vi "DKGSM_old.vi"(9 "input":T1, 10 "State":string) -> (2 "DKGSMOutput":T2)   [LabVIEW 2015]
uses:
  Typedefs/DKGSMOut.ctl
  Typedefs/DKGSMin.ctl
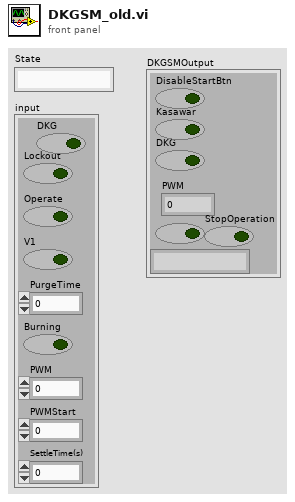
[diagram p1: front panel]
types:
  T1 = typedef "DKGSMin.ctl" = cluster{"Lockout":bool, "Operate":bool, "V1":bool, "PurgeTime":dbl, "Burning":bool, "PWM":i32, "PWMStart":i32, "SettleTime(s)":dbl, "DKG":bool}
  T2 = typedef "DKGSMOut.ctl" = cluster{"DisableStartBtn":bool, "Kasawar":bool, "DKG":bool, "PWM":i32, "Purge":bool, "Opis":string, "StopOperation":bool}
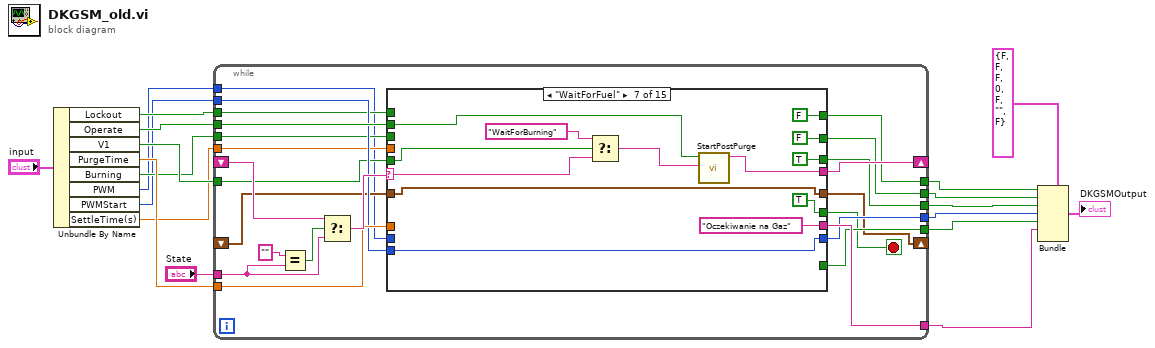
[diagram p0: block diagram]
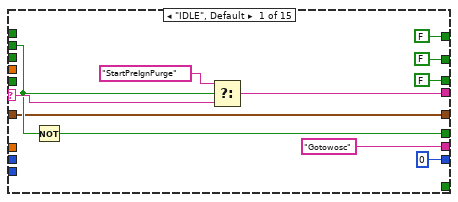
[diagram p2: hidden frame]
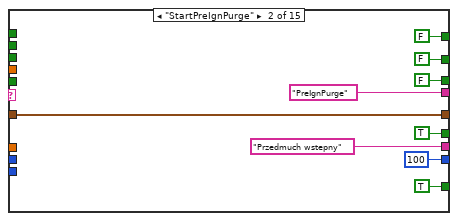
[diagram p3: hidden frame]
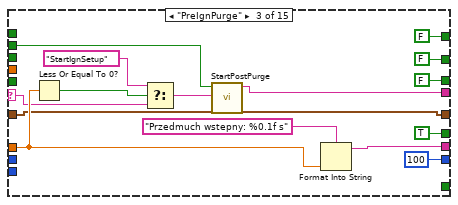
[diagram p4: hidden frame]
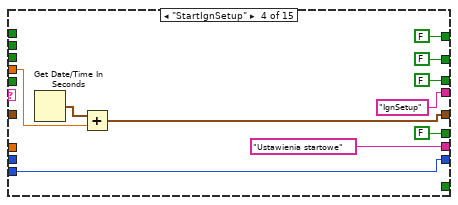
[diagram p5: hidden frame]
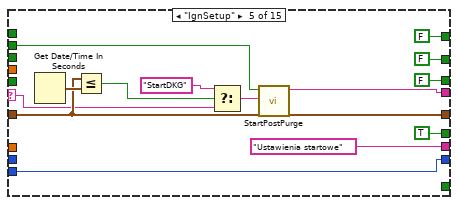
[diagram p6: hidden frame]
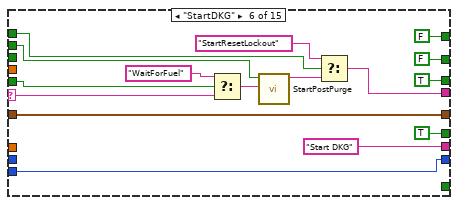
[diagram p7: hidden frame]
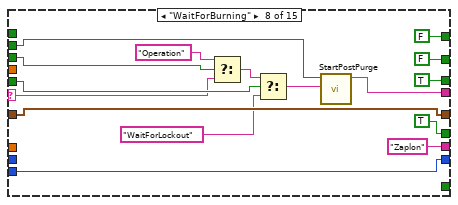
[diagram p8: hidden frame]
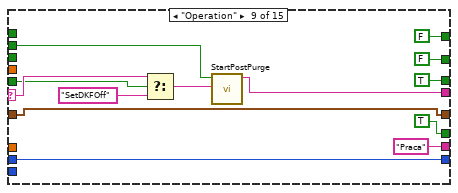
[diagram p9: hidden frame]
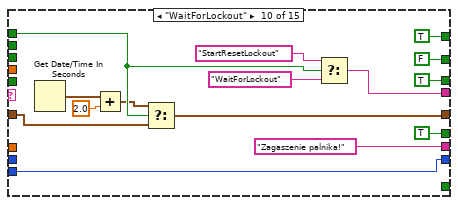
[diagram p10: hidden frame]
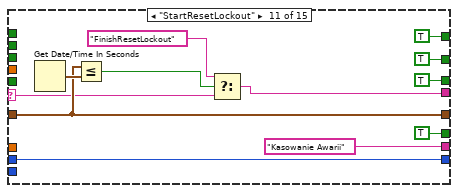
[diagram p11: hidden frame]
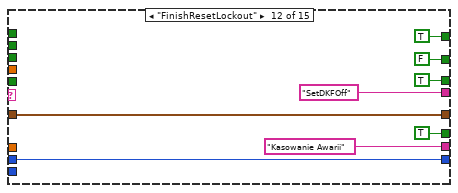
[diagram p12: hidden frame]
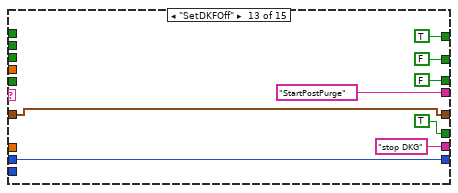
[diagram p13: hidden frame]
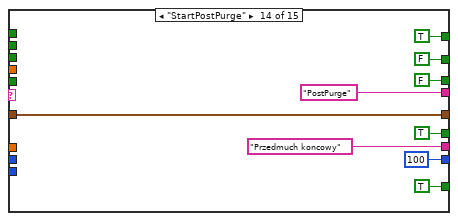
[diagram p14: hidden frame]
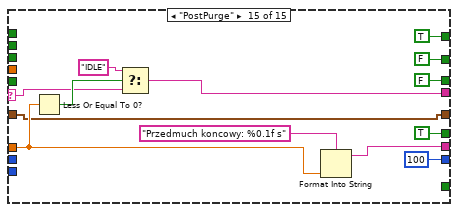
[diagram p15: hidden frame]
diagram:
  n1 = Unbundle By Name("input") -> ("Lockout"=w8:bool, "Operate"=w7:bool, "V1"=w6:bool, "PurgeTime"=w5:dbl, "Burning"=w4:bool, "PWM"=w3:i32, "PWMStart"=w2:i32, "SettleTime(s)"=w1:dbl)
  n2 = while {
    tunnel: "State" -> [w39]
    shift-right: [w36] -> _
    shift-left: _ -> [w40]
    tunnel: w7 -> [w35]
    tunnel: [w34] -> w12
    tunnel: w5 -> [w33]
    tunnel: [w32] -> w13
    tunnel: w2 -> [w31]
    tunnel: [w30] -> w14
    tunnel: w1 -> [w28]
    shift-right: [w27] -> _
    shift-left: _ -> [w26]
    tunnel: w8 -> [w25]
    tunnel: w6 -> [w24]
    tunnel: [w23] -> w15
    tunnel: w4 -> [w22]
    tunnel: w3 -> [w21]
    tunnel: [w20] -> w16
    tunnel: [w19] -> w17
    stop <- w29 stop-if-true
    n3 = Equal?(x="", y=w39) -> (x = y?=w41:bool)
    n4 = Select(t=w40, s=w41, f=w39) -> (s? t:f=w37:string)
    n5 = case shown="\"WaitForFuel\"" w37 {
      selector: w37 -> [w52 _ w70 _ w92 w107 w117 w131 w151 _ w180 _ _ _ w219]
      tunnel: [w51 "PreIgnPurge" ("t") w75 "IgnSetup" ("t") w95 w109 w124 w140 w157 w167 w178 "SetDKFOff" ("f") "StartPostPurge" ("f") "PostPurge" ("t") w218] -> w36
      tunnel: w35 -> [w47 _ w76 _ w94 w113 w123 w139 w156 _ _ _ _ _ _]
      tunnel: ["Gotowosc" "Przedmuch wstepny" w73 "Ustawienia startowe" "Ustawienia startowe" "Start DKG" "Oczekiwanie na Gaz" "Zaplon" "Praca" "Zagaszenie palnika!" "Kasowanie Awarii" "Kasowanie Awarii" "stop DKG" "Przedmuch koncowy" w222] -> w34
      tunnel: w33 -> [_ _ w72 _ _ _ _ _ _ _ _ _ _ _ w221]
      tunnel: [_ TRUE _ _ _ _ _ _ _ _ _ _ _ TRUE _] -> w32
      tunnel: w31 -> [_ _ _ w86 w100 w114 w126 w142 _ w171 _ _ _ _ _]
      tunnel: [0 ("PWMStart") 100 ("PWMStart") 100 ("PWMStart") w86 w100 w114 w126 w142 w154 w171 w175 w190 w198 100 ("PWMStart") 100 ("PWMStart")] -> w30
      tunnel: [w48 TRUE TRUE FALSE TRUE TRUE TRUE TRUE TRUE TRUE TRUE TRUE TRUE TRUE TRUE] -> w29
      tunnel: w28 -> [_ _ _ w84 _ _ _ _ _ _ _ _ _ _ _]
      tunnel: [w46 w57 w66 w83 w96 w116 w129 w145 w158 w161 w182 w193 w201 w206 w215] -> w27
      tunnel: w26 -> [w46 w57 w66 _ w96 w116 w129 w145 w158 w162 w182 w193 w201 w206 w215]
      tunnel: w25 -> [_ _ _ _ _ w112 _ _ _ w166 _ _ _ _ _]
      tunnel: w24 -> [_ _ _ _ _ w108 w118 w138 w148 _ _ _ _ _ _]
      tunnel: [FALSE FALSE FALSE FALSE FALSE TRUE TRUE TRUE TRUE TRUE TRUE TRUE FALSE FALSE FALSE] -> w23
      tunnel: w22 -> [_ _ _ _ _ _ _ w136 _ _ _ _ _ _ _]
      tunnel: w21 -> [_ _ _ _ _ _ _ _ w154 _ w175 w190 w198 _ _]
      tunnel: [FALSE FALSE FALSE FALSE FALSE FALSE FALSE FALSE FALSE FALSE TRUE FALSE FALSE FALSE FALSE] -> w20
      tunnel: [FALSE FALSE FALSE FALSE FALSE FALSE FALSE FALSE FALSE TRUE TRUE TRUE TRUE TRUE TRUE] -> w19
      frame "IDLE", Default {
        n6 = Not(x=w47) -> (.not. x?=w48:bool)
        n7 = Select(t="StartPreIgnPurge", s=w47, f=w52) -> (s? t:f=w51:string)
      }
      frame "StartPreIgnPurge" {
      }
      frame "PreIgnPurge" {
        n8 = Less Or Equal To 0?(x=w72) -> (x <= 0?=w71:bool)
        n9 = Select(t="StartIgnSetup", s=w71, f=w70) -> (s? t:f=w69:string)
        n10 = call "StartPostPurge.vi"("t"=w69, "Operate"=w76) -> ("f"=w75:string)  [unwired: 9 in]
        n11 = Format Into String(format string="Przedmuch wstepny: %0.1f s", w72) -> (resulting string=w73:string)  [unwired: 2 in, 1 out]
      }
      frame "StartIgnSetup" {
        n12 = Get Date/Time In Seconds() -> (seconds since 1Jan1904=w85:timestamp)
        n13 = Add(x=w85, y=w84) -> (x+y=w83:timestamp)
      }
      frame "IgnSetup" {
        n14 = Get Date/Time In Seconds() -> (seconds since 1Jan1904=w97:timestamp)
        n15 = Less Or Equal?(x=w96, y=w97) -> (x <= y?=w93:bool)
        n16 = Select(t="StartDKG", s=w93, f=w92) -> (s? t:f=w90:string)
        n17 = call "StartPostPurge.vi"("t"=w90, "Operate"=w94) -> ("f"=w95:string)  [unwired: 9 in]
      }
      frame "StartDKG" {
        n18 = Select(t="WaitForFuel", s=w108, f=w107) -> (s? t:f=w105:string)
        n19 = call "StartPostPurge.vi"("t"=w105, "Operate"=w113) -> ("f"=w111:string)  [unwired: 9 in]
        n20 = Select(t="StartResetLockout", s=w112, f=w111) -> (s? t:f=w109:string)
      }
      frame "WaitForFuel" {
        n21 = Select(t="WaitForBurning", s=w118, f=w117) -> (s? t:f=w122:string)
        n22 = call "StartPostPurge.vi"("t"=w122, "Operate"=w123) -> ("f"=w124:string)  [unwired: 9 in]
      }
      frame "WaitForBurning" {
        n23 = Select(t="Operation", s=w136, f=w131) -> (s? t:f=w135:string)
        n24 = Select(t=w135, s=w138, f="WaitForLockout") -> (s? t:f=w137:string)
        n25 = call "StartPostPurge.vi"("t"=w137, "Operate"=w139) -> ("f"=w140:string)  [unwired: 9 in]
      }
      frame "Operation" {
        n26 = Select(t=w151, s=w148, f="SetDKFOff") -> (s? t:f=w150:string)
        n27 = call "StartPostPurge.vi"("t"=w150, "Operate"=w156) -> ("f"=w157:string)  [unwired: 9 in]
      }
      frame "WaitForLockout" {
        n28 = Get Date/Time In Seconds() -> (seconds since 1Jan1904=w165:timestamp)
        n29 = Add(x=w165, y=2.0) -> (x+y=w163:timestamp)
        n30 = Select(t=w163, s=w166, f=w162) -> (s? t:f=w161:timestamp)
        n31 = Select(t="StartResetLockout", s=w166, f="WaitForLockout") -> (s? t:f=w167:string)
      }
      frame "StartResetLockout" {
        n32 = Get Date/Time In Seconds() -> (seconds since 1Jan1904=w183:timestamp)
        n33 = Less Or Equal?(x=w182, y=w183) -> (x <= y?=w181:bool)
        n34 = Select(t="FinishResetLockout", s=w181, f=w180) -> (s? t:f=w178:string)
      }
      frame "FinishResetLockout" {
      }
      frame "SetDKFOff" {
      }
      frame "StartPostPurge" {
      }
      frame "PostPurge" {
        n35 = Less Or Equal To 0?(x=w221) -> (x <= 0?=w220:bool)
        n36 = Select(t="IDLE", s=w220, f=w219) -> (s? t:f=w218:string)
        n37 = Format Into String(format string="Przedmuch koncowy: %0.1f s", w221) -> (resulting string=w222:string)  [unwired: 2 in, 1 out]
      }
    }
  }
  n38 = Bundle(cluster=T2 {"DisableStartBtn"=FALSE, "Kasawar"=FALSE, "DKG"=FALSE, "PWM"=0, "Purge"=FALSE, "Opis"="", "StopOperation"=FALSE} ("output cluster"), "DisableStartBtn"=w17, "Kasawar"=w16, "DKG"=w15, "PWM"=w14, "Purge"=w13, "Opis"=w12) -> (→"DKGSMOutput":T2)  [unwired: 1 in]
